vi "Bind Blob.vi"(8 "error in (no error)":errorcluster, 10 "Blob":string, 11 "SQL Statement in":refnum<class "SQL Statement.lvclass">) -> (0 "error out":errorcluster, 3 "SQL Statement out":refnum<class "SQL Statement.lvclass">)   [LabVIEW 2023, in "SQLiteSupport.lvlib" / "SQL Statement.lvclass"]
doc: "Binds the next parameter as an SQLite3 BLOB datatype."
uses:
  SQL Statement.lvclass
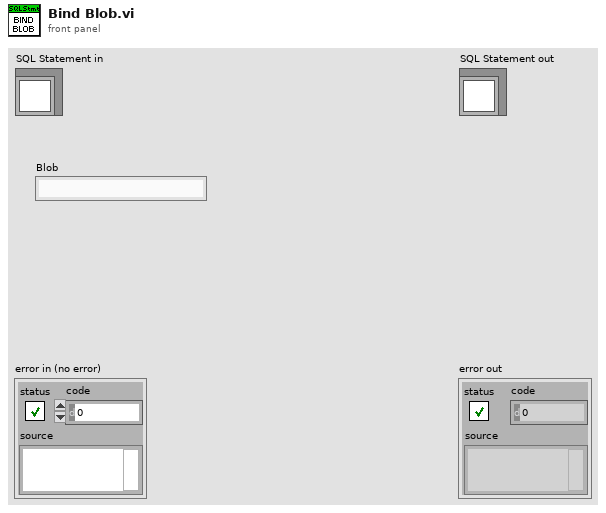
[diagram p1: front panel]
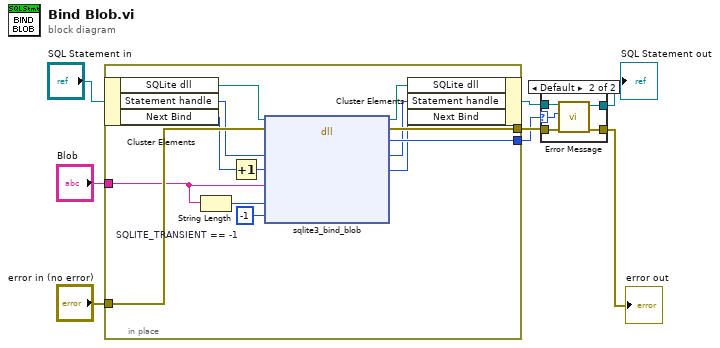
[diagram p0: block diagram]
diagram:
  n1 = in-place {
    in-place-border: "error in (no error)" -> [w21]
    in-place-border: "Blob" -> [w19]
    in-place-border: [w17] -> w6
    in-place-border: [w16] -> w5
    w20 = i64 -1  # SQLITE_TRANSIENT == -1
    n2 = in-place-cluster #1("SQL Statement in") -> ("SQLite dll"=w12:path, "Statement handle"=w13:u64, "Next Bind"=w14:i32)
    n3 = String Length(string=w19) -> (length=w18:i32)
    n4 = Increment(x=w14) -> (x+1=w15:i32)
    n5 = dll-call lib="C:/LabVIEW_JDP/Support/SQLite/sqlite3.dll" fn="sqlite3_bind_blob"(path in=w12, error in=w21, "Statement"=w13, "Parameter"=w15, "Blob"=w19, "Number of Bytes"=w18, "arg5"=w20) -> (path out=w11:path, error out=w17:errorcluster, "Result Code"=w16:i32, "Statement"=w10:u64, "Parameter"=w9:i32)  [unwired: 4 in]
    n6 = in-place-cluster #1("SQLite dll"=w11, "Statement handle"=w10, "Next Bind"=w9) -> (w1:refnum<class "SQL Statement.lvclass">)
  }
  n7 = case shown="Default" w5 {
    selector: w5 -> [_ w25]
    tunnel: [w22 w28] -> w4
    tunnel: w6 -> [w23 w27]
    tunnel: [w23 w26] -> w3
    tunnel: w1 -> [w22 w24]
    frame 0 {
      # "No Error"
    }
    frame Default {
      n8 = call "Error Message.vi"("error in (no error)"=w27, "error code"=w25, "SQL Statement In"=w24) -> ("error out"=w26:errorcluster, "SQL Statement Out"=w28:refnum<class "SQL Statement.lvclass">)  [unwired: 7 in]
    }
  }
  "error out" <- w3
  "SQL Statement out" <- w4
